vi "Amp lin scan.vi"(9 "Gain %/s":fxp<+/-,64,32>, 10 "Amp inc/dec":u8[](array[numeric]), 11 "Gain":fxp<+,32,4>[](array[numeric])) -> (3 "Array":fxp<+,32,4>[](array[numeric]))   [LabVIEW 2020]
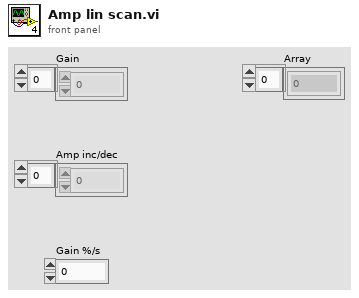
[diagram p1: front panel]
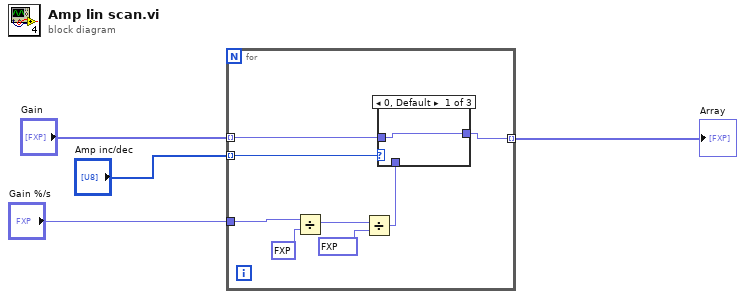
[diagram p0: block diagram]
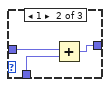
[diagram p2: hidden frame]
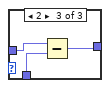
[diagram p3: hidden frame]
diagram:
  n1 = for {
    tunnel: "Gain" -> [w10] mode=indexing
    tunnel: "Gain %/s" -> [w8]
    tunnel: [w5] -> w3 mode=indexing
    tunnel: "Amp inc/dec" -> [w6] mode=indexing
    n2 = Divide(x=w8, y=fxp<+,5,7> 100.0) -> (x/y=w9:fxp<+/-,64,32>)
    n3 = Divide(x=w9, y=fxp<+,20,5> 30.303009033203125) -> (x/y=w12:fxp<+/-,64,32>)
    n4 = case shown="0, Default" w6 {
      tunnel: w10 -> [w13 w16 w19]
      tunnel: [w13 w15 w17] -> w5
      tunnel: w12 -> [_ w14 w18]
      frame 0, Default {
      }
      frame 1 {
        n5 = Add(x=w16, y=w14) -> (x+y=w15:fxp<+,32,4>)
      }
      frame 2 {
        n6 = Subtract(x=w19, y=w18) -> (x-y=w17:fxp<+,32,4>)
      }
    }
  }
  "Array" <- w3
